vi "Convert to betta.vi"(0 "Ro %":dbl format="%#_7g") -> (10 "Ro betta":dbl)   [LabVIEW 2023]
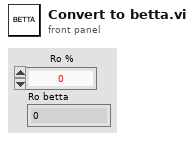
[diagram p1: front panel]
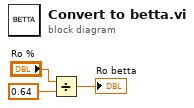
[diagram p0: block diagram]
diagram:
  n1 = Divide(x="Ro %", y=0.64) -> (x/y=→"Ro betta":dbl)
